vi "MPM_Get_Unit.vi"(8 "error in (no error)":errorcluster, 11 ".NET Reference in":refnum<k24>) -> (0 "error out":errorcluster, 2 "unit":enum16{"dBmA, dBm", "mW, mA"}(ring), 3 "Reference out":refnum<k24>)   [LabVIEW 2017]
doc: "get setting unit"
uses:
  LV_IL_Sample/DLL/InstrumentDLL.dll
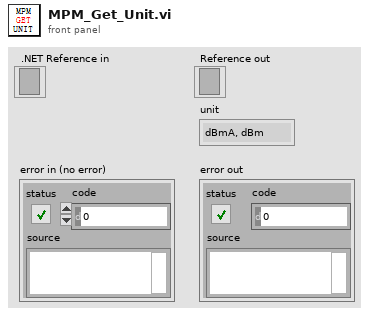
[diagram p1: front panel]
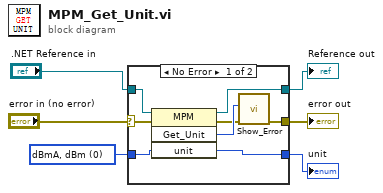
[diagram p0: block diagram]
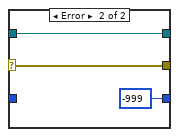
[diagram p2: hidden frame]
diagram:
  w3 = 0 items=["dBmA, dBm", "mW, mA"] ("unit")
  n1 = case shown="No Error" "error in (no error)" {
    selector: "error in (no error)" -> [w7 w17]
    tunnel: [w14 -999 ("unit")] -> w6
    tunnel: ".NET Reference in" -> [w13 w15]
    tunnel: [w12 w15] -> w4
    tunnel: w3 -> [w11 _]
    tunnel: [w8 w17] -> w2
    frame No Error {
      n2 = invoke on="调用节点" class="MPM" method="Get_Unit"(reference=w13, error in=w7, "unit"=w11) -> (reference out=w12:refnum<k24>, error out=w9:errorcluster, "Get_Unit"=w10:i32, "unit"=w14:i32)  [unwired: 1 in]
      n3 = call "Show_Error.vi"("error in (no error)"=w9, "Error"=w10) -> ("error out"=w8:errorcluster)  [unwired: 9 in]
    }
    frame Error {
    }
  }
  "Reference out" <- w4
  "error out" <- w2
  "unit" <- w6
